vi "Read Measurement Data (Raw NChan).vi"(0 "VISA resource name":refnum<visa-resource-name>, 5 "Start Channel (1)":string="0001", 7 "End Channel (1)":string="0001", 11 "error in (no error)":errorcluster) -> (2 "Date Time":timestamp=timestamp(3345116400 s since 1904-01-01) format="%<%H:%M:%S%3u\n%x>T", 4 "VISA resource name out":refnum<visa-resource-name>, 6 "Channel":string[](array[string]), 8 "Data":i32[](array[numeric]), 10 "Data Status":i32[](array[ring]) items=["Normal", "Differential Input", "Skip", "Over", "Error", "Burnout", "Power Failure"], 13 "Alarm Status":i32[][](array[ring]) items=["No Alarm", "High Limit Alarm (H)", "Low Limit Alarm (L)", "Difference High Limit Alarm (h)", "Difference Low Limit Alarm (l)", "High Limit on Rate-of-change Alarm (R)", "Low Limit on Rate-of-change Alarm (r)", "Delay High Limit Alarm (T)", "Delay Low Limit Alarm (t)"], 14 "Data Type":i32[](array[ring]) items=["NULL", "INT", "FLOAT"], 15 "error out":errorcluster)   [LabVIEW 2020, in "Yokogawa GX Series.lvlib"]
doc: "This VI reads the raw measurement data by Binary."
uses:
  <instrlib>/Yokogawa GX Series/Yokogawa GX Series.lvlib
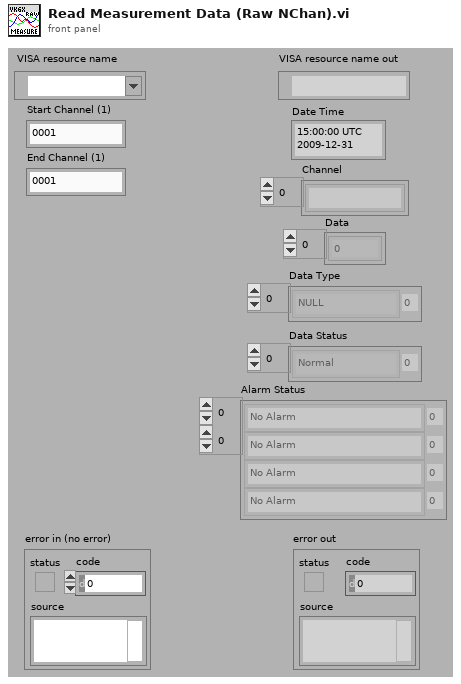
[diagram p1: front panel]
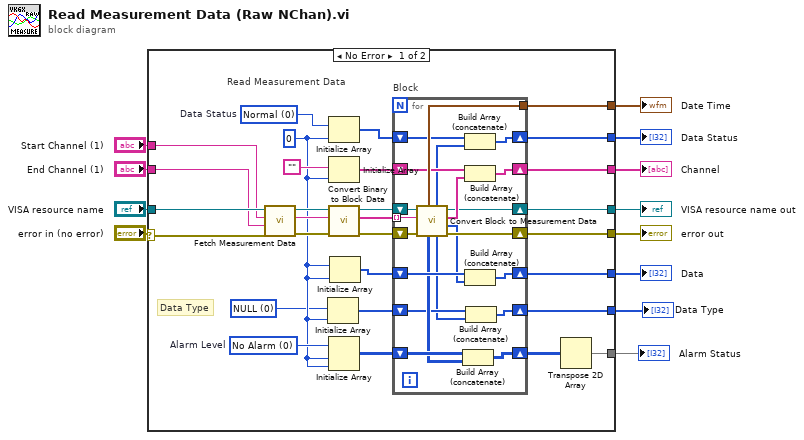
[diagram p0: block diagram]
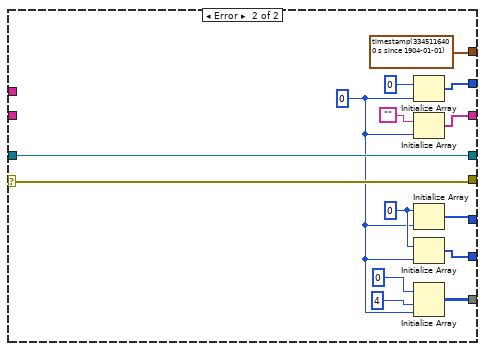
[diagram p2: hidden frame]
diagram:
  n1 = case shown="No Error" "error in (no error)" {
    selector: "error in (no error)" -> [w17 w75]
    tunnel: "VISA resource name" -> [w41 w76]
    tunnel: [w40 w76] -> w11
    tunnel: [w39 w75] -> w10
    tunnel: [w38 timestamp(3345116400 s since 1904-01-01)] -> w9
    tunnel: [w37 w70] -> w8
    tunnel: [w36 w69] -> w7
    tunnel: [w35 w68] -> w6
    tunnel: [w34 w72] -> w5
    tunnel: "End Channel (1)" -> [w33 _]
    tunnel: "Start Channel (1)" -> [w32 _]
    tunnel: [w13 w63] -> w1
    frame No Error {
      w15 = 0 items=["NULL", "INT", "FLOAT"]
      w21 = 0 items=["No Alarm", "High Limit Alarm (H)", "Low Limit Alarm (L)", "Difference High Limit Alarm (h)", "Difference Low Limit Alarm (l)", "High Limit on Rate-of-change Alarm (R)", "Low Limit on Rate-of-change Alarm (r)", "Delay High Limit Alarm (T)", "Delay Low Limit Alarm (t)"]  # Alarm Level
      w22 = 0 items=["Normal", "Differential Input", "Skip", "Over", "Error", "Burnout", "Power Failure"]  # Data Status
      w16 = 0 ("Channel Number")
      # "Data Type"
      # "Read Measurement Data"
      n2 = call <instrlib>:"Fetch Measurement Data.vi"("error in (no error)"=w17, "End Channel (1)"=w33, "Start Channel (1)"=w32, "VISA resource name"=w41) -> ("error out"=w26:errorcluster, "Measurement Data"=w28:string, "VISA resource name out"=w27:refnum<visa-resource-name>)  [unwired: 1 in, 4 out]
      n3 = Initialize Array(w15, w16) -> (w14:i32[])
      n4 = Initialize Array(w22, w16) -> (w24:i32[])
      n5 = Initialize Array("", w16) -> (w20:string[])
      n6 = call <instrlib>:"Convert Binary to Block Data.vi"("error in (no error)"=w26, "Measurement Binary Data (\"\")"=w28, "VISA resource name"=w27) -> ("error out"=w30:errorcluster, "Measurement Block Data"=w29:string[], "VISA resource name out"=w31:refnum<visa-resource-name>)  [unwired: 6 out]
      n7 = Initialize Array(w21, w16, w16) -> (w23:i32[][])
      n8 = Initialize Array(w16, w16) -> (w18:i32[])
      n9 = for "Block" {
        shift-right: [w47] -> w39
        shift-left: w30 -> [w62]
        tunnel: w29 -> [w61] mode=indexing
        tunnel: [w59] -> w38
        shift-right: [w56] -> w37
        shift-left: w20 -> [w58]
        shift-right: [w54] -> w36
        shift-left: w18 -> [w55]
        shift-right: [w52] -> w34
        shift-left: w24 -> [w53]
        shift-right: [w49] -> w25
        shift-left: w23 -> [w51]
        shift-right: [w48] -> w40
        shift-left: w31 -> [w60]
        shift-right: [w42] -> w13
        shift-left: w14 -> [w44]
        n10 = call <instrlib>:"Convert Block to Measurement Data.vi"("error in (no error)"=w62, "Measurement Block Data (\"\")"=w61, "VISA resource name"=w60) -> ("error out"=w47:errorcluster, "Data"=w46:i32[], "Channel"=w57:string[], "VISA resource name out"=w48:refnum<visa-resource-name>, "Data Type"=w43:i32[], "Data Status"=w45:i32[], "Alarm Status"=w50:i32[][], "Date Time"=w59:timestamp)  [unwired: 1 out]
        n11 = Build Array (concatenate)(w51, w50) -> (w49:i32[][])
        n12 = Build Array (concatenate)(w53, w45) -> (w52:i32[])
        n13 = Build Array (concatenate)(w58, w57) -> (w56:string[])
        n14 = Build Array (concatenate)(w55, w46) -> (w54:i32[])
        n15 = Build Array (concatenate)(w44, w43) -> (w42:i32[])
      }
      n16 = Transpose 2D Array(2D array=w25) -> (transposed array=w35:i32[][])
    }
    frame Error {
      w64 = 0
      w65 = 0
      n17 = Initialize Array(0, w64) -> (w72:i32[])
      n18 = Initialize Array("", w64) -> (w70:string[])
      n19 = Initialize Array(w65, w64) -> (w69:i32[])
      n20 = Initialize Array(w65, w64) -> (w63:i32[])
      n21 = Initialize Array(0, 4, w64) -> (w68:i32[][])
    }
  }
  "error out" <- w10
  "VISA resource name out" <- w11
  "Channel" <- w8
  "Alarm Status" <- w6
  "Date Time" <- w9
  "Data" <- w7
  "Data Status" <- w5
  "Data Type" <- w1
